vi "tools_createNewITaskClass.vi"   [LabVIEW 2023]
types:
  T1 = typedef "stopMechanismType.ctl" = enum16{"BooleanNotifier", "BooleanUE", "MsgUE"}
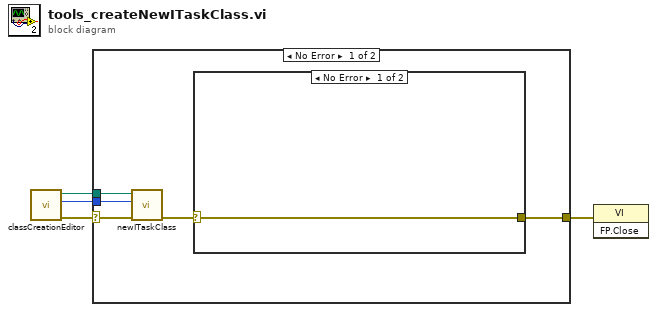
[diagram p0: block diagram]
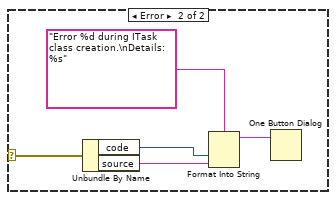
[diagram p2: hidden frame]
diagram:
  n1 = call "classCreationEditor.vi"() -> ("error out"=w3:errorcluster, "stopMechanismType"=w1:T1, "classPath"=w4:path)  [unwired: 9 in]
  n2 = case shown="No Error" w3 {
    selector: w3 -> [w8 _]
    tunnel: w4 -> [w9 _]
    tunnel: [w6 _] -> w2
    tunnel: w1 -> [w5 _]
    frame No Error {
      n3 = call "newITaskClass.vi"("error in (no error)"=w8, "stopMechanismType"=w5, "classPath"=w9) -> ("error out"=w7:errorcluster)  [unwired: 7 in, 1 out]
      n4 = case shown="No Error" w7 {
        selector: w7 -> [w10 w13]
        tunnel: [w10 _] -> w6
        frame No Error {
        }
        frame Error {
          n5 = Unbundle By Name(w13) -> ("code"=w12:i32, "source"=w11:string)
          n6 = Format Into String(format string="Error %d during ITask class creation.\nDetails: %s", w12, w11) -> (resulting string=w14:string)  [unwired: 2 in, 1 out]
          n7 = One Button Dialog(message=w14) -> ()  [unwired: 1 in, 1 out]
        }
      }
    }
    frame Error {
    }
  }
  n8 = invoke class="VI" method="FP.Close"(error in=w2) -> ()  [unwired: 2 in, 3 out]
